vi "reas_ios_file.vi"() -> ()   [LabVIEW 2012]
panel:
  out "size (in bytes)":i64=29677869
  out "ofset in":i64=29677868
  out "Numeric":i32=723840
  out "offset out":i64=29677860
  in  "frame":i64(slide) scale=0.0..11881.0
  in  "file (use dialog)":path=path "\\\\IFMB-02-024B-10\\Ischemia2/IOS/2019-06-03/2019-06-03_15-58-53.ios"
  in  "stop":bool
  out "Image":T1(plugin-control)
  in  "X size":i32=696
  out "IOS":u16[](array[numeric])
  in  "Y size":i32=520
  out "data":string
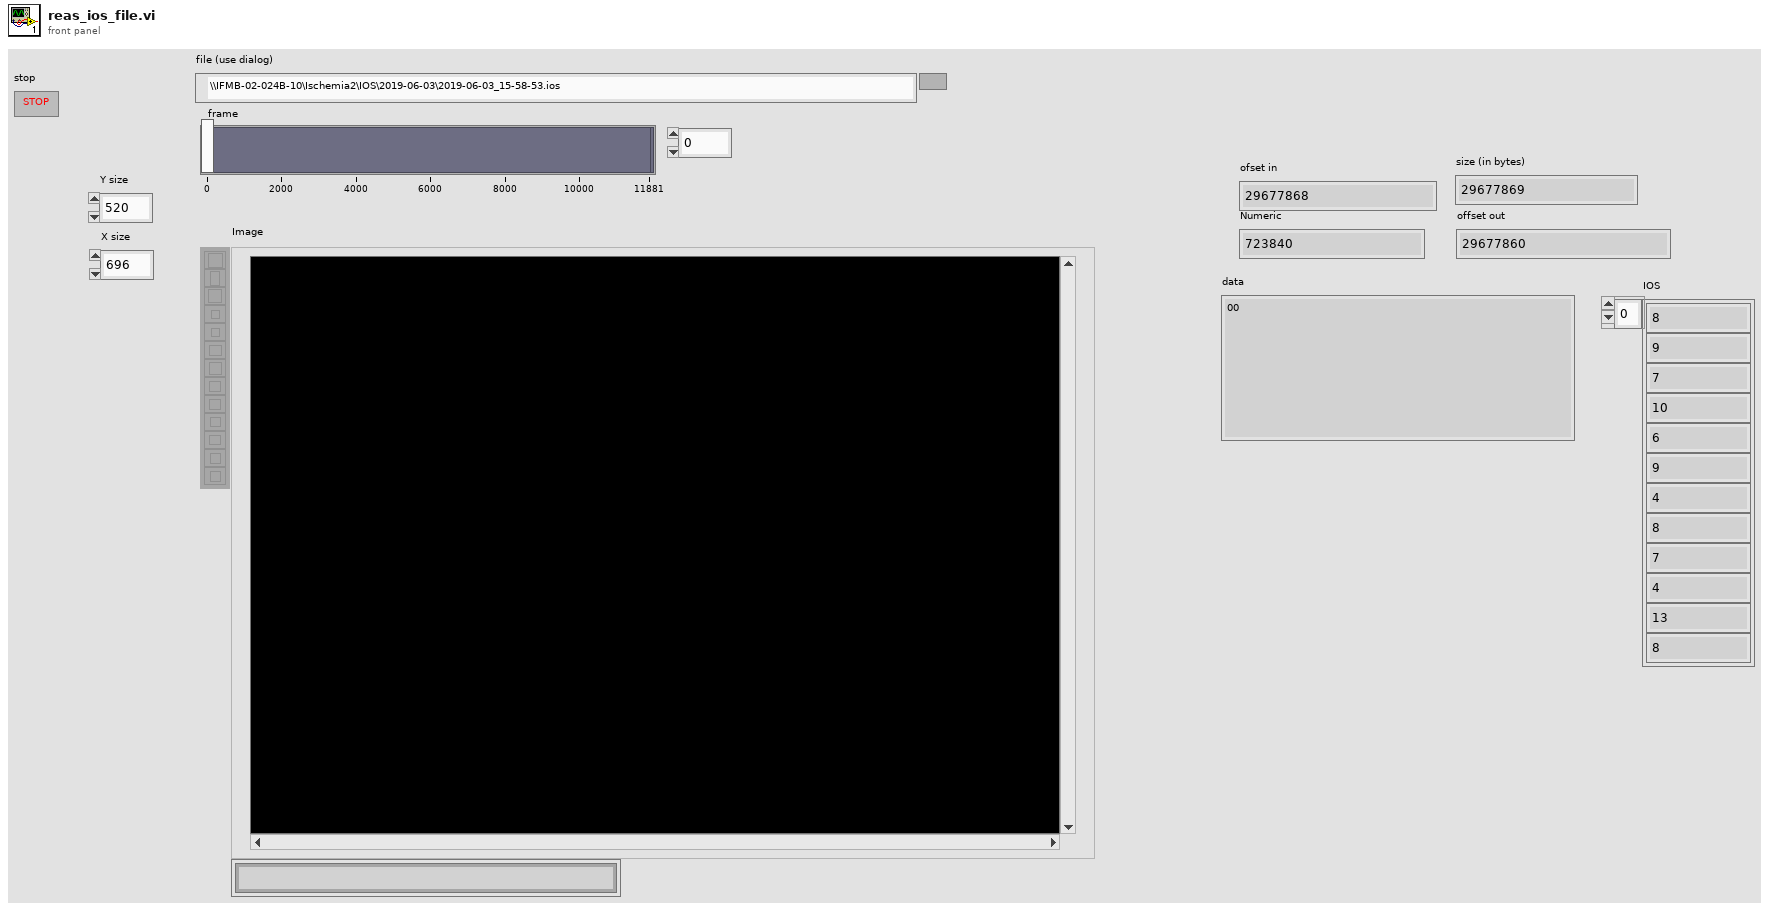
[diagram p1: front panel]
types:
  T1 = typedef "IMAQ Image.ctl" = refnum<image>
  T2 = typedef "Image Type" = u32
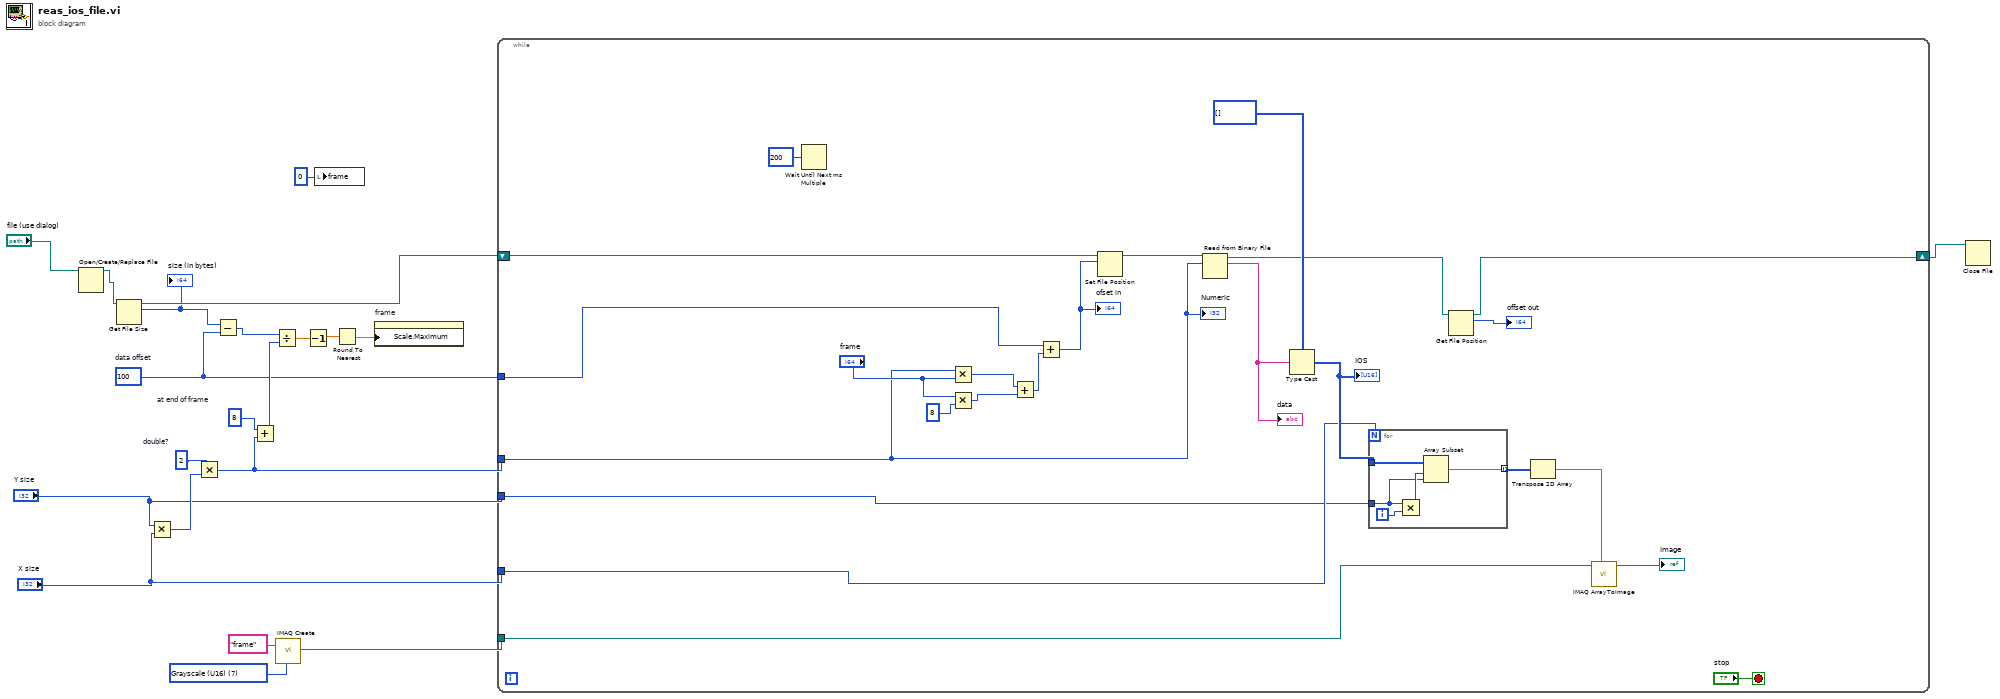
[diagram p0: block diagram]
diagram:
  w6 = i64 100  # data offset
  w11 = 8  # at end of frame
  w16 = 2  # double?
  w19 = T2 7 items=["Grayscale (U8)", "Grayscale (I16)", "Grayscale (SGL)", "Complex (CSG)", "RGB (U32)", "HSL (U32)", "RGB (U64)", "Grayscale (U16)"] ("Image Type")
  n1 = Open/Create/Replace File(file path (use dialog)="file (use dialog)") -> (refnum out=w13:refnum<file>)  [unwired: 5 in, 2 out]
  n2 = Get File Size(file=w13) -> (refnum out=w12:refnum<file>, size (in bytes)=w7:i64)  [unwired: 1 in, 1 out]
  "size (in bytes)" <- w7
  n3 = Multiply(x="Y size", y="X size") -> (x*y=w15:i32)
  n4 = Multiply(x=w16, y=w15) -> (x*y=w10:i32)
  n5 = Subtract(x=w7, y=w6) -> (x-y=w5:i64)
  n6 = Add(x=w11, y=w10) -> (x+y=w9:i32)
  n7 = Divide(x=w5, y=w9) -> (x/y=w4:dbl)
  n8 = call "IMAQ Create"("Image Name"="frame", "Image Type"=w19) -> ("New Image"=w17:T1)  [unwired: 3 in, 1 out]
  n9 = Decrement(x=w4) -> (x-1=w3:dbl)
  n10 = local write "frame"(i64 0 ("frame")) -> ()
  n11 = Round To Nearest(number=w3) -> (nearest integer value=w2:dbl)
  n12 = property on="frame" class="Slide (strict)"("Scale.Maximum"=w2) -> ()  [unwired: 2 in, 2 out]
  n13 = while {
    shift-right: [w24] -> w20
    shift-left: w12 -> [w32]
    tunnel: w17 -> [w31]
    tunnel: w10 -> [w26]
    tunnel: "X size" -> [w30]
    tunnel: "Y size" -> [w29]
    tunnel: w6 -> [w22]
    stop <- "stop" stop-if-true
    n14 = Wait Until Next ms Multiple(millisecond multiple=u32 200) -> ()  [unwired: 1 out]
    n15 = Multiply(x=w26, y="frame") -> (x*y=w33:i64)
    n16 = Multiply(x="frame", y=i64 8) -> (x*y=w34:i64)
    n17 = Add(x=w33, y=w34) -> (x+y=w36:i64)
    n18 = Add(x=w22, y=w36) -> (x+y=w27:i64)
    "ofset in" <- w27
    n19 = Set File Position(offset (in bytes) (0)=w27, refnum=w32) -> (refnum out=w44:refnum<file>)  [unwired: 2 in, 1 out]
    n20 = Read from Binary File(10:w26, 11:w44) -> (2:w43:string, 3:w25:refnum<file>)  [unwired: 4 in, 2 out]
    "data" <- w43
    n21 = Type Cast(type=u16[] [], x=w43) -> (*(type *) &x=w40:u16[])
    "IOS" <- w40
    n22 = for {
      N: w30 -> [_]
      tunnel: w40 -> [w50]
      tunnel: [w49] -> w39 mode=indexing
      tunnel: w29 -> [w46]
      i -> [w48]
      n23 = Multiply(x=w46, y=w48) -> (x*y=w47:i32)
      n24 = Array Subset(array=w50, index=w47, length=w46) -> (w49:u16[])
    }
    n25 = Get File Position(7:w25) -> (2:→"offset out":i64, 3:w24:refnum<file>)  [unwired: 1 in, 1 out]
    n26 = Transpose 2D Array(2D array=w39) -> (transposed array=w37:u16[][])
    n27 = call "IMAQ ArrayToImage"("Image Pixels (U16)"=w37, "Image"=w31) -> ("Image Out"=→"Image":T1)  [unwired: 8 in, 1 out]
    "Numeric" <- w26
  }
  n28 = Close File(refnum=w20) -> ()  [unwired: 1 in, 2 out]
